vi "Terminals From Types.vi"(11 "Types":T4[](array[typedef])) -> (3 "Terminals":T1[](array[typedef]))   [LabVIEW 2022 SP3, in "FlexBlocks Support.lvlib"]
uses:
  FlexBlocks Support.lvlib
  Terminal State.ctl
  Terminal Status.ctl
  Terminal Direction.ctl
  Terminal Draw Style.ctl
  Special Terminal.ctl
  Value Mode.ctl
  Type Descriptor.ctl
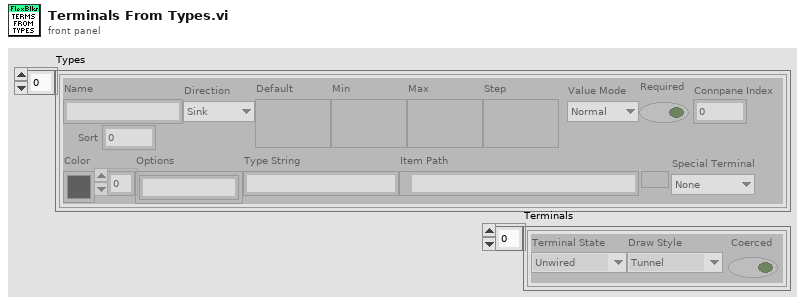
[diagram p1: front panel]
types:
  T1 = typedef "FlexBlocks Support.lvlib/Terminal Status.ctl" = cluster{"Terminal State":T2, "Draw Style":T3, "Coerced":bool}
  T2 = typedef "FlexBlocks Support.lvlib/Terminal State.ctl" = enum16{"Unwired", "BadType", "BadRef", "Channel", "Value", "Control Ref"}
  T3 = typedef "FlexBlocks Support.lvlib/Terminal Draw Style.ctl" = enum16{"Tunnel", "BadType", "BadRef", "Channel", "Value", "Control Ref"}
  T4 = typedef "FlexBlocks Support.lvlib/Type Descriptor.ctl" = cluster{"Name":string, "Direction":T5, "Default":variant, "Min":variant, "Max":variant, "Step":variant, "Value Mode":T6, "Color":u32, "Options":string[], "Type String":string, "Item Path":path, "Required":bool, "Connpane Index":i32, "Special Terminal":T7, "Sort":i32}
  T5 = typedef "FlexBlocks Support.lvlib/Terminal Direction.ctl" = enum16{"Sink", "Source"}
  T6 = typedef "FlexBlocks Support.lvlib/Value Mode.ctl" = enum16{"Normal", "Range", "Select"}
  T7 = typedef "FlexBlocks Support.lvlib/Special Terminal.ctl" = enum16{"None", "Action", "Init", "Tag", "State in", "State out", "Error"}
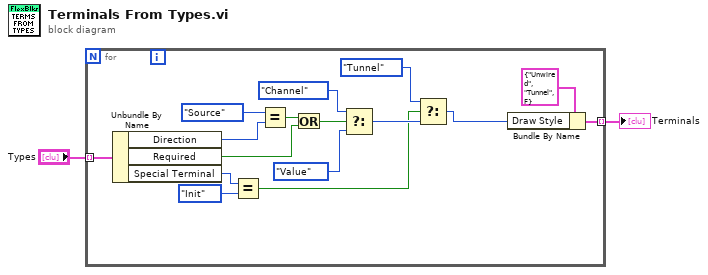
[diagram p0: block diagram]
diagram:
  n1 = for {
    tunnel: "Types" -> [w18] mode=indexing
    tunnel: [w11] -> w1 mode=indexing
    n2 = Unbundle By Name(w18) -> ("Direction"=w17:T5, "Required"=w14:bool, "Special Terminal"=w10:T7)
    n3 = Equal?(x=w10, y=Special_Terminal."Init") -> (x = y?=w6:bool)
    n4 = Equal?(x=Terminal_Direction."Source", y=w17) -> (x = y?=w15:bool)
    n5 = Or(x=w15, y=w14) -> (x .or. y?=w12:bool)
    n6 = Select(t=Terminal_Draw_Style."Channel" ("Draw Style"), s=w12, f=Terminal_Draw_Style."Value" ("Draw Style")) -> (s? t:f=w8:T3)
    n7 = Select(t=Terminal_Draw_Style."Tunnel" ("Draw Style"), s=w6, f=w8) -> (s? t:f=w7:T3)
    n8 = Bundle By Name(cluster=T1 {"Terminal State"=enum."Unwired", "Draw Style"=enum."Tunnel", "Coerced"=FALSE} ("Terminal Status"), "Draw Style"=w7) -> (w11:T1)
  }
  "Terminals" <- w1
